vi "CanControlSetAccFilter.vi"(4 "extended":bool, 5 "error in":errorcluster {"code" format="%.0x"}, 6 "Mask":u32 format="%032b", 7 "Code":u32 format="%032b", 8 "CAN Control Handle in":u32 format="%x") -> (0 "error out":errorcluster {"code" format="%.0x"}, 3 "CAN Control Handle out":u32)   [LabVIEW 2011]
doc: "Sets the global acceptance filter of the CAN controller."
uses:
  vcilva.dll
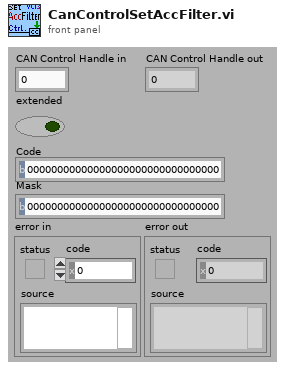
[diagram p1: front panel]
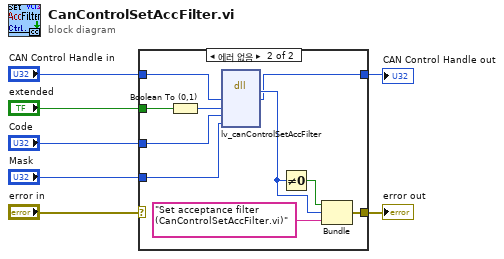
[diagram p0: block diagram]
diagram:
  n1 = case shown="에러 없음" "error in" {
    selector: "error in" -> [w9 _]
    tunnel: [w9 w19] -> w6
    tunnel: "CAN Control Handle in" -> [w8 w15]
    tunnel: [w8 w14] -> w4
    tunnel: "Code" -> [_ w13]
    tunnel: "Mask" -> [_ w12]
    tunnel: "extended" -> [_ w10]
    frame Error {
    }
    frame No Error {
      n2 = Boolean To (0,1)(Boolean=w10) -> (0, 1=w11:i16)
      n3 = dll-call lib="vcilva.dll" fn="lv_canControlSetAccFilter"("hCanCtl"=w15, "fExtend"=w11, "dwCode"=w13, "dwMask"=w12) -> (w16:i32, "hCanCtl"=w14:u32)  [unwired: 6 in, 2 out]
      n4 = Not Equal To 0?(x=w16) -> (x != 0?=w18:bool)
      n5 = Bundle(w18, w16, "Set acceptance filter (CanControlSetAccFilter.vi)") -> (w19:errorcluster)  [unwired: 1 in]
    }
  }
  "error out" <- w6
  "CAN Control Handle out" <- w4
